vi "HVPulseTiming.vi"(0 "Strings in":string[](array[string])=["C:\\CuspControl\\GPIB and Network\\Cusp\\HVPulseTiming.txt", "6723"], 1 "Dubs in":dbl[](array[numeric])=[1.2e-05, 1.3e-06]) -> ()   [LabVIEW 2018]
panel:
  in  "Pulse Delay (s)":dbl=1.2e-05
  in  "file (use dialog)":path=path "C:/CuspControl/GPIB and Network/Cusp/HVPulseTiming.txt"
  out "x-y":u32=1
  in  "Pulse Width (s)":dbl=1.3e-06 format="%_4p"
  in  "subvi":bool=TRUE
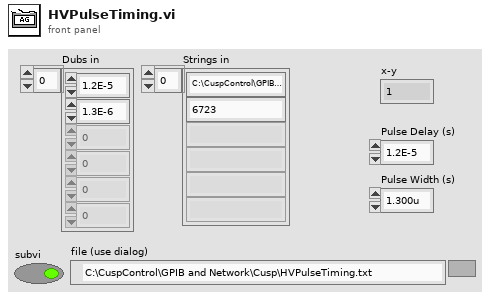
[diagram p1: front panel]
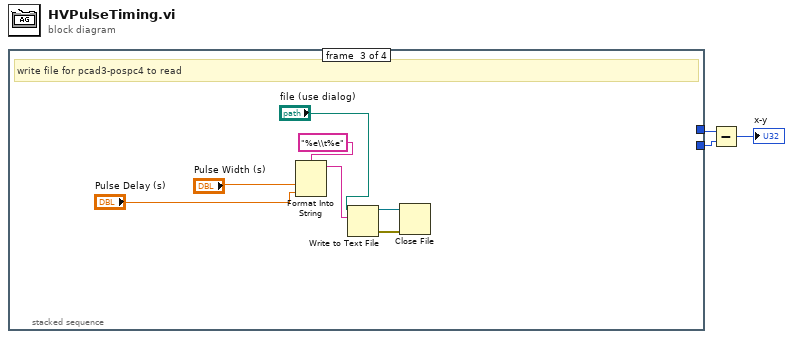
[diagram p0: block diagram]
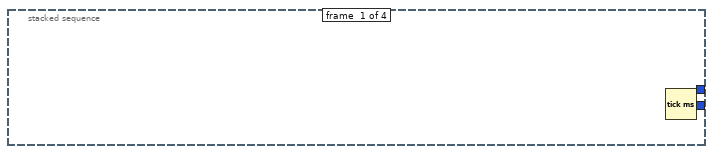
[diagram p2: hidden frame]
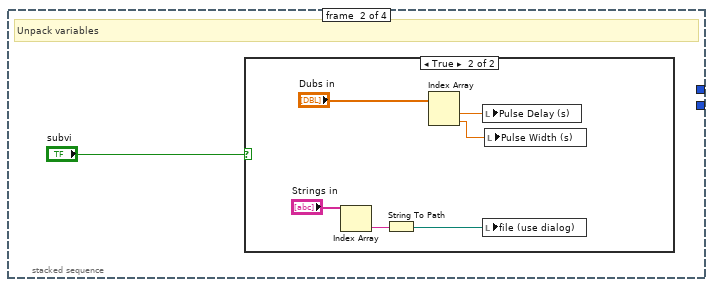
[diagram p3: hidden frame]
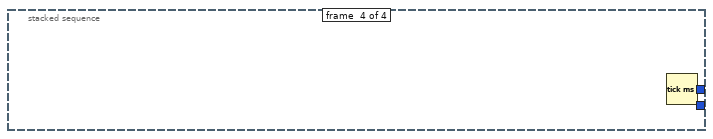
[diagram p5: hidden frame]
diagram:
  n1 = stacked-sequence {
    tunnel: [w4 _ _ _] -> w3
    tunnel: [_ _ _ w19] -> w2
    frame #0 {
      n2 = Tick Count (ms)() -> (millisecond timer value=w4:u32)
    }
    frame #1 {
      # "Unpack variables"
      n3 = case shown="True" "subvi" {
        frame False {
        }
        frame True {
          n4 = Index Array(array="Strings in") -> (element=w8:string)  [unwired: 1 in]
          n5 = String To Path(string=w8) -> (path=w7:path)
          n6 = Index Array(array="Dubs in") -> (element #1=w9:dbl, element #2=w6:dbl)  [unwired: 2 in]
          n7 = local write "Pulse Delay (s)"(w9) -> ()
          n8 = local write "file (use dialog)"(w7) -> ()
          n9 = local write "Pulse Width (s)"(w6) -> ()
        }
      }
    }
    frame #2 {
      # "write file for pcad3-pospc4 to read"
      n10 = Format Into String(format string="%e\\t%e", "Pulse Width (s)", "Pulse Delay (s)") -> (resulting string=w16:string)  [unwired: 2 in, 1 out]
      n11 = Write to Text File(file (use dialog)="file (use dialog)", text=w16) -> (refnum out=w17:refnum<file>, error out=w18:errorcluster)  [unwired: 2 in, 1 out]
      n12 = Close File(refnum=w17, error in=w18) -> ()  [unwired: 2 out]
    }
    frame #3 {
      n13 = Tick Count (ms)() -> (millisecond timer value=w19:u32)
    }
  }
  n14 = Subtract(x=w2, y=w3) -> (x-y=→"x-y":u32)
